vi "Evaluate Car Position.vi"(8 "error in (no error)":errorcluster, 11 "Car Position Monitor Model in":refnum<class "Simulated Car Position Monitor Model.lvclass">) -> (0 "error out":errorcluster, 3 "Car Position Monitor Model out":refnum<class "Simulated Car Position Monitor Model.lvclass">)   [LabVIEW 2019, in "Simulated Car Position Monitor Model.lvclass"]
uses:
  <vilib>/gpm_packages/@cs/Car-wash/Source/Simulated Car Position Monitor Model/Simulated Car Position Monitor Model.lvclass
  C:/Program Files/National Instruments/LabVIEW 2019/vi.lib/gpm_packages/@cs/Car-wash/Source/iCar Position Monitor Model/iCar Position Monitor Model/iCar Position Monitor Model.lvclass
  <vilib>/gpm_packages/@cs/Car-wash/Source/Simulated Car Position Monitor Model/Simulated Car Position Monitor Model.lvclass/Simulated Car Position Monitor Model.ctl
  <vilib>/gpm_packages/@cs/Car-wash/Source/iCar Position Monitor Model/iCar Position Monitor Model/iCar Position Monitor Model.lvclass
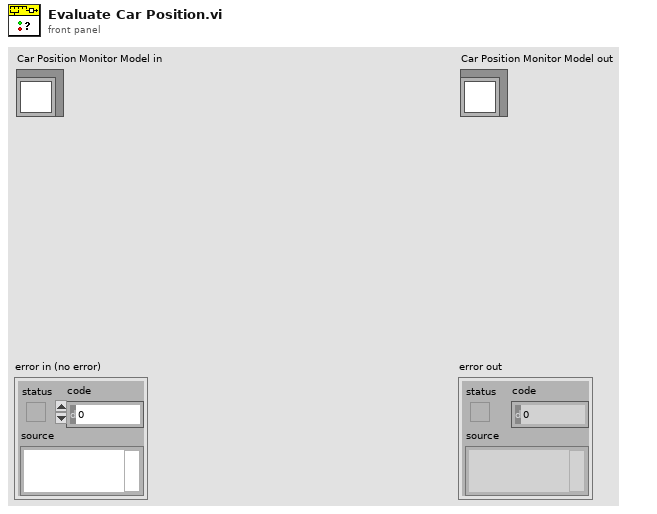
[diagram p1: front panel]
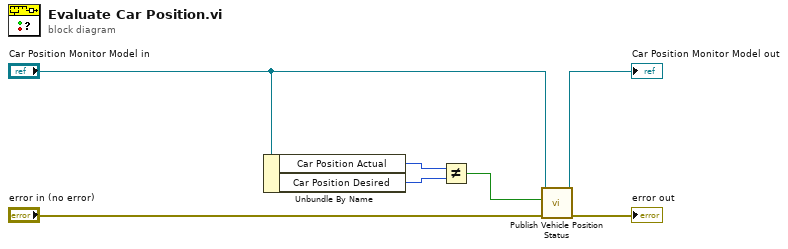
[diagram p0: block diagram]
diagram:
  n1 = Unbundle By Name("Car Position Monitor Model in") -> ("Car Position Actual"=w3:u8, "Car Position Desired"=w2:u8)
  n2 = Not Equal?(x=w3, y=w2) -> (x != y?=w1:bool)
  n3 = call <vilib>:"Publish Vehicle Position Status.vi"("error in (no error)"="error in (no error)", "Vehicle Out of Position"=w1, "iCar Position Monitor Model in"="Car Position Monitor Model in") -> ("error out"=→"error out":errorcluster, "iCar Position Monitor Model out"=→"Car Position Monitor Model out":refnum<class "Simulated Car Position Monitor Model.lvclass">)  [unwired: 7 in]
